vi "SetSyncDivider.vi"(8 "error in (no error)":errorcluster, 10 "SyncDivider":i32(ring)=1 items=["1"=1, "2"=2, "4"=4, "8"=8, "16"=16], 11 "Multiharp in":refnum<class "Multiharp.lvclass">) -> (0 "error out":errorcluster, 3 "Multiharp out":refnum<class "Multiharp.lvclass">)   [LabVIEW 2023, in "Multiharp.lvlib" / "Multiharp.lvclass"]
uses:
  Multiharp.lvclass
  <vilib>/ActorFramework/Actor/Actor.lvclass
  Multiharp Messages/SetSyncTrigger Msg/SetSyncTrigger Msg.lvclass
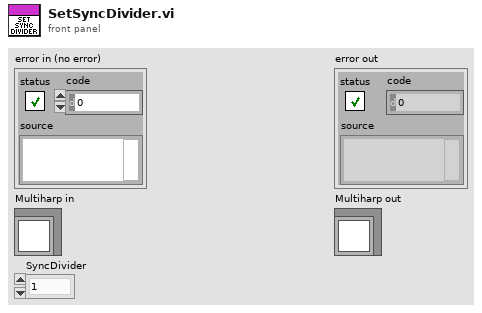
[diagram p1: front panel]
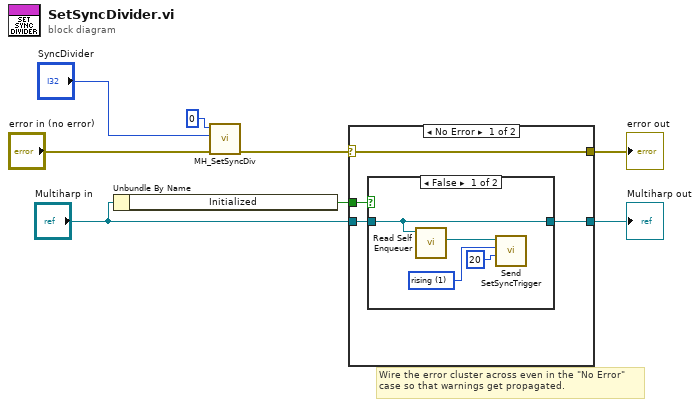
[diagram p0: block diagram]
diagram:
  # "Wire the error cluster across even in the \"No Error\"\ncase so that warnings get propagated."
  n1 = Unbundle By Name("Multiharp in") -> ("Initialized"=w8:bool)
  n2 = call "MH_SetSyncDiv.vi"("error in (no error)"="error in (no error)", "SyncDivider"="SyncDivider", "devidx"=0) -> ("error out"=w5:errorcluster)  [unwired: 7 in, 1 out]
  n3 = case shown="No Error" w5 {
    selector: w5 -> [w9 w18]
    tunnel: w8 -> [w12 _]
    tunnel: "Multiharp in" -> [w11 w19]
    tunnel: [w10 w19] -> w2
    tunnel: [w9 w18] -> w4
    frame No Error {
      n4 = case shown="False" w12 {
        tunnel: w11 -> [w16 w17]
        tunnel: [w16 w17] -> w10
        frame False {
          w14 = 1 items=["falling", "rising"] ("SyncEdge")
          n5 = call <vilib>:"Read Self Enqueuer.vi"("Actor"=w16) -> ("Self Enqueuer"=w15:refnum<class "Message Enqueuer.lvclass">)  [unwired: 10 in]
          n6 = call "Send SetSyncTrigger.vi"("SyncLevel"=20, "SyncEdge"=w14, "Message Enqueuer"=w15) -> ()  [unwired: 7 in, 2 out]
        }
        frame True {
          # "Send message to UI"
        }
      }
    }
    frame Error {
    }
  }
  "error out" <- w4
  "Multiharp out" <- w2
